vi "Coerce Trigger Coupling.vi"(8 "error in (no error)":errorcluster, 11 "5105 in":refnum<class "5105.lvclass">) -> (0 "error out":errorcluster, 3 "5105 out":refnum<class "5105.lvclass">)   [LabVIEW 2019, in "5105.lvlib" / "5105.lvclass"]
uses:
  5105.lvclass
  C:/Users/rdexter/Documents/Development/Drivers/PPL/Oscilloscope.lvlibp/Oscilloscope.lvclass
  builds/Instruments/Oscilloscope.lvlibp/Custom Controls/Trigger Coupling.ctl
  builds/Instruments/Oscilloscope.lvlibp/Accessors/Read Trigger Settings.vi
  builds/Instruments/Oscilloscope.lvlibp/Accessors/Write Trigger Settings.vi
  builds/Instruments/Oscilloscope.lvlibp/Oscilloscope.lvclass
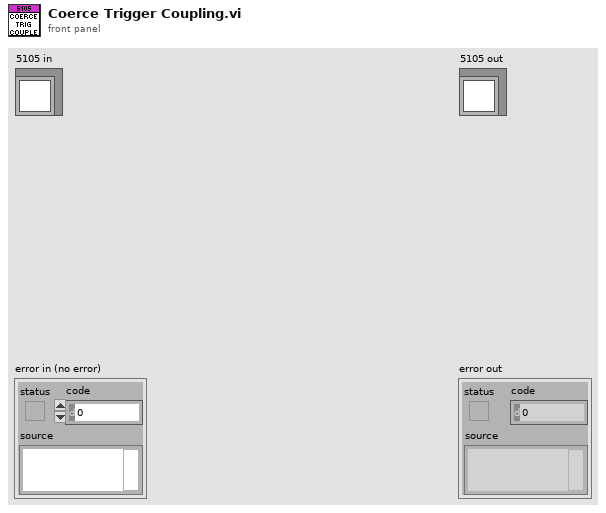
[diagram p1: front panel]
types:
  T1 = typedef "Oscilloscope.lvlibp/Oscilloscope.lvclass/Trigger Coupling.ctl" = u16
  T2 = typedef "Oscilloscope.lvlibp/Oscilloscope.lvclass/Trigger Settings.ctl" = cluster{"Edge:":T3, "Level":dbl, "Source":T4, "trigger coupling":T1, "Holdoff":dbl, "Delay":dbl, "Trigger Modifier":T5, "Trigger Type":T6}
  T3 = typedef "Oscilloscope.lvlibp/Oscilloscope.lvclass/Edge Select.ctl" = u16
  T4 = typedef "Oscilloscope.lvlibp/Oscilloscope.lvclass/Channel List.ctl" = u16
  T5 = typedef "Oscilloscope.lvlibp/Oscilloscope.lvclass/Trigger Modifier.ctl" = enum16{"Invalid_Setting", "None", "Auto Trigger"}
  T6 = typedef "Oscilloscope.lvlibp/Oscilloscope.lvclass/Trigger Type.ctl" = enum16{"Immediate", "Analog Edge", "Digital", "Window", "Hysteresis"}
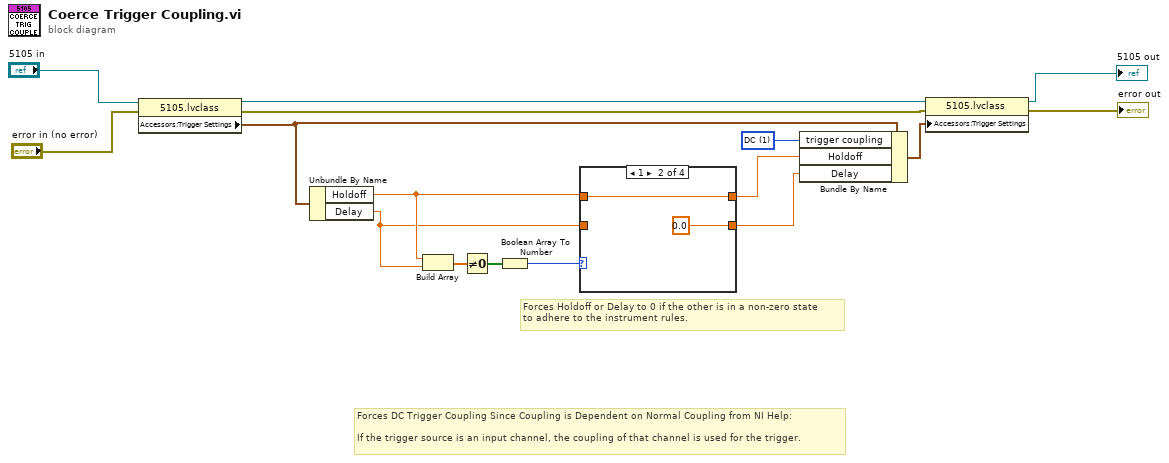
[diagram p0: block diagram]
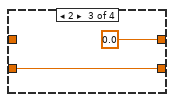
[diagram p3: hidden frame]
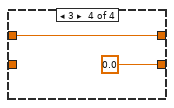
[diagram p4: hidden frame]
diagram:
  w10 = T1 1 items=["AC", "DC", "HF Reject", "LF Reject", "AC Plus HF Reject"] ("trigger coupling")
  # "Forces Holdoff or Delay to 0 if the other is in a non-zero state\nto adhere to the instrument rules."
  # "Forces DC Trigger Coupling Since Coupling is Dependent on Normal Coupling from NI Help:\n\nIf the trigger source is an input channel, the coupling of that channel is used for the trigger."
  n1 = property class="5105.lvclass"(reference="5105 in", error in="error in (no error)") -> (reference out=w9:refnum<class "5105.lvclass">, error out=w14:errorcluster, "Accessors:Trigger Settings"=w8:T2)
  n2 = Unbundle By Name(w8) -> ("Holdoff"=w4:dbl, "Delay"=w3:dbl)
  n3 = Build Array(w4, w3) -> (w7:dbl[])
  n4 = Not Equal To 0?(x=w7) -> (x != 0?=w6:bool[])
  n5 = Boolean Array To Number(Boolean array=w6) -> (number=w5:u32)
  n6 = case shown="1" w5 {
    tunnel: w4 -> [w18 w20 _ w24]
    tunnel: w3 -> [w17 _ w22 _]
    tunnel: [w18 w20 0.0 ("Holdoff") w24] -> w2
    tunnel: [w17 0.0 ("Delay") w22 0.0 ("Delay")] -> w1
    frame 0, Default {
    }
    frame 1 {
    }
    frame 2 {
    }
    frame 3 {
    }
  }
  n7 = Bundle By Name(cluster=w8, "trigger coupling"=w10, "Holdoff"=w2, "Delay"=w1) -> (w11:T2)
  n8 = property class="5105.lvclass"(reference=w9, error in=w14, "Accessors:Trigger Settings"=w11) -> (reference out=→"5105 out":refnum<class "5105.lvclass">, error out=→"error out":errorcluster)
